vi "write shared memory.vi"(6 "channel classification":T1, 8 "error in":errorcluster, 10 "data table":T2, 11 "module in":refnum<class "Shared Memory runtime.lvclass">) -> (0 "error out":errorcluster, 2 "data table out":T2, 3 "module out":refnum<class "Shared Memory runtime.lvclass">)   [LabVIEW 2014, in "Shared Memory runtime.lvclass"]
uses:
  Shared Memory runtime.lvclass
  <vilib>/NI/Tag Bus/table/data table.ctl
  <vilib>/NI/Tag Bus Module Framework/channel/channel classification.ctl
  Shared Memory runtime.lvclass/Shared Memory runtime.ctl
  <vilib>/NI/Tag Bus/table/data polymorphs/read many/read Doubles.vi
  <vilib>/NI/NI Linux RT IPC/Shared Memory/Pointer Operations/Write 1D Array DBL.vi
  <vilib>/NI/Tag Bus/table/data polymorphs/read many/read Singles.vi
  <vilib>/NI/NI Linux RT IPC/Shared Memory/Pointer Operations/Write 1D Array SGL.vi
  <vilib>/NI/Tag Bus/table/data polymorphs/read many/read I64s.vi
  <vilib>/NI/NI Linux RT IPC/Shared Memory/Pointer Operations/Write 1D Array I64.vi
  <vilib>/NI/Tag Bus/table/data polymorphs/read many/read I32s.vi
  <vilib>/NI/NI Linux RT IPC/Shared Memory/Pointer Operations/Write 1D Array I32.vi
  <vilib>/NI/Tag Bus/table/data polymorphs/read many/read I16s.vi
  <vilib>/NI/NI Linux RT IPC/Shared Memory/Pointer Operations/Write 1D Array I16.vi
  <vilib>/NI/Tag Bus/table/data polymorphs/read many/read I8s.vi
  <vilib>/NI/NI Linux RT IPC/Shared Memory/Pointer Operations/Write 1D Array I8.vi
  <vilib>/NI/Tag Bus/table/data polymorphs/read many/read U64s.vi
  <vilib>/NI/NI Linux RT IPC/Shared Memory/Pointer Operations/Write 1D Array U64.vi
  <vilib>/NI/Tag Bus/table/data polymorphs/read many/read U32s.vi
  <vilib>/NI/NI Linux RT IPC/Shared Memory/Pointer Operations/Write 1D Array U32.vi
  <vilib>/NI/Tag Bus/table/data polymorphs/read many/read U16s.vi
  <vilib>/NI/NI Linux RT IPC/Shared Memory/Pointer Operations/Write 1D Array U16.vi
  <vilib>/NI/Tag Bus/table/data polymorphs/read many/read U8s.vi
  <vilib>/NI/NI Linux RT IPC/Shared Memory/Pointer Operations/Write 1D Array U8.vi
  <vilib>/NI/Tag Bus/table/data polymorphs/read many/read Booleans.vi
  <vilib>/NI/NI Linux RT IPC/Shared Memory/Pointer Operations/Write 1D Array Boolean.vi
  <vilib>/NI/Tag Bus/table/data polymorphs/read sequential/read sequential Doubles.vi
  <vilib>/NI/Tag Bus/table/data polymorphs/read sequential/read sequential Singles.vi
  <vilib>/NI/Tag Bus/table/data polymorphs/read sequential/read sequential I64s.vi
  <vilib>/NI/Tag Bus/table/data polymorphs/read sequential/read sequential I32s.vi
  <vilib>/NI/Tag Bus/table/data polymorphs/read sequential/read sequential I16s.vi
  <vilib>/NI/Tag Bus/table/data polymorphs/read sequential/read sequential I8s.vi
  <vilib>/NI/Tag Bus/table/data polymorphs/read sequential/read sequential U64s.vi
  <vilib>/NI/Tag Bus/table/data polymorphs/read sequential/read sequential U32s.vi
  <vilib>/NI/Tag Bus/table/data polymorphs/read sequential/read sequential U16s.vi
  <vilib>/NI/Tag Bus/table/data polymorphs/read sequential/read sequential U8s.vi
  <vilib>/NI/Tag Bus/table/data polymorphs/read sequential/read sequential Booleans.vi
  Read input data.vi
  Read processing parameters.vi
  Read processing results.vi
  Read output data.vi
  <vilib>/NI/NI Linux RT IPC/Shared Memory/Classes/Shared Memory/Shared Memory.lvclass
  <vilib>/NI/Tag Bus/table/data table.lvlib
  <vilib>/NI/NI Linux RT IPC/Shared Memory/Linux RT IPC.Shared Memory.lvlib
  <vilib>/NI/Tag Bus Module Framework/channel/TBM channel.lvclass
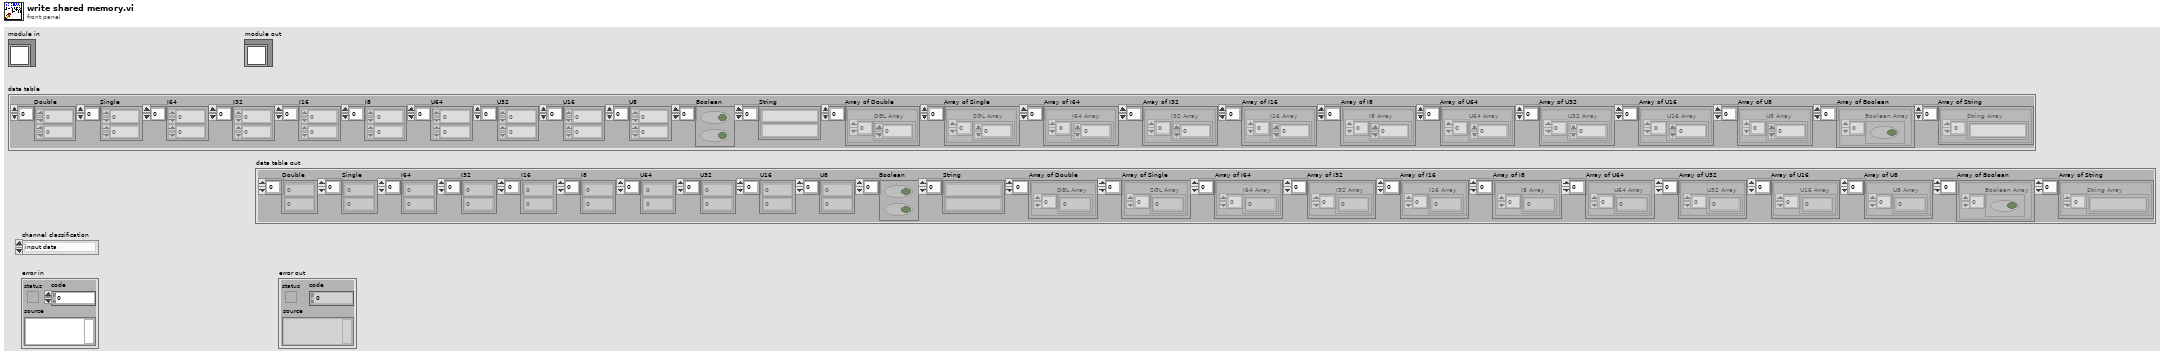
[diagram p1: front panel]
types:
  T1 = typedef "TBM channel.lvclass/channel classification.ctl" = enum16{"input data", "output data", "processing parameter", "processing result"}
  T2 = typedef "tag bus.lvlib/data table.lvlib/data table.ctl" = cluster{"Double":dbl[], "Single":sgl[], "I64":i64[], "I32":i32[], "I16":i16[], "I8":i8[], "U64":u64[], "U32":u32[], "U16":u16[], "U8":u8[], "Boolean":bool[], "String":string[], "Array of Double":cluster{"DBL Array":dbl[]}[], "Array of Single":cluster{"SGL Array":sgl[]}[], "Array of I64":cluster{"I64 Array":i64[]}[], "Array of I32":cluster{"I32 Array":i32[]}[], "Array of I16":cluster{"I16 Array":i16[]}[], "Array of I8":cluster{"I8 Array":i8[]}[], "Array of U64":cluster{"U64 Array":u64[]}[], "Array of U32":cluster{"U32 Array":u32[]}[], "Array of U16":cluster{"U16 Array":u16[]}[], "Array of U8":cluster{"U8 Array":u8[]}[], "Array of Boolean":cluster{"Boolean Array":bool[]}[], "Array of String":cluster{"String Array":string[]}[]}
  T3 = typedef "Shared Memory runtime.lvclass/channel runtime.ctl" = cluster{"channel classification":T1, "data type":T4, "pointer to shared memory":u64, "number of elements":u64, "data dictionary index":cluster{i32[]}, "shared memory":T5, "first tag index":i32, "sequential tags?":bool}
  T4 = typedef "tag bus.lvlib/tag descriptor.lvclass/Data Type.ctl" = enum16{"Double", "Single", "I64", "I32", "I16", "I8", "U64", "U32", "U16", "U8", "Boolean", "String", "Array of Double", "Array of Single", "Array of I64", "Array of I32", "Array of I16", "Array of I8", "Array of U64", "Array of U32", "Array of U16", "Array of U8", "Array of Boolean", "Array of String"}
  T5 = typedef "Linux RT IPC.Shared Memory.lvlib/reference.ctl" = refnum<data-value>
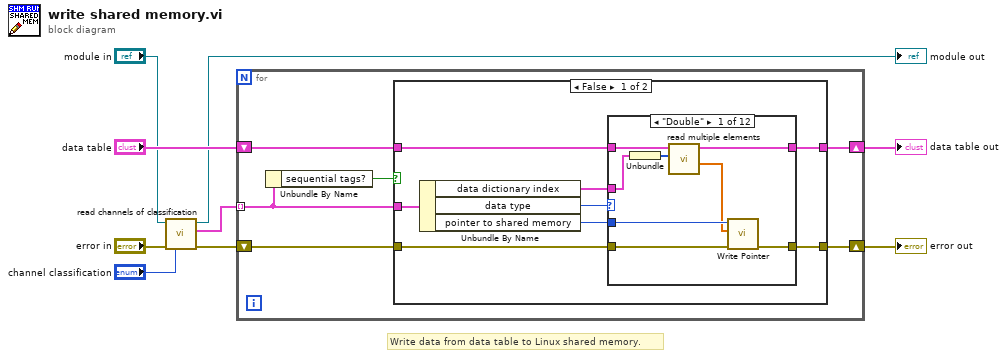
[diagram p0: block diagram]
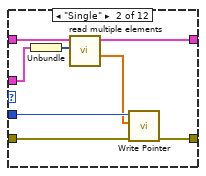
[diagram p2: hidden frame]
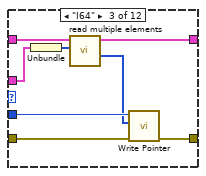
[diagram p3: hidden frame]
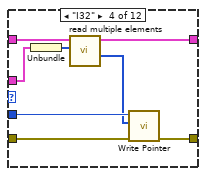
[diagram p4: hidden frame]
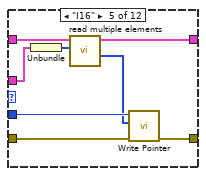
[diagram p5: hidden frame]
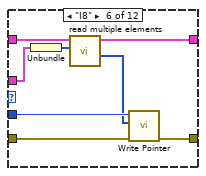
[diagram p6: hidden frame]
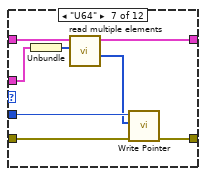
[diagram p7: hidden frame]
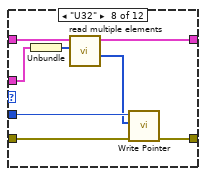
[diagram p8: hidden frame]
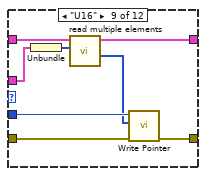
[diagram p9: hidden frame]
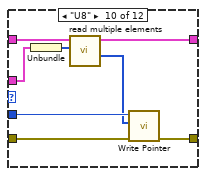
[diagram p10: hidden frame]
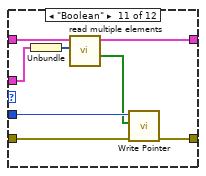
[diagram p11: hidden frame]
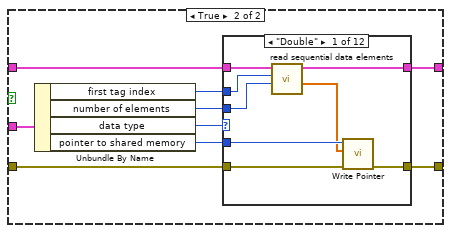
[diagram p13: hidden frame]
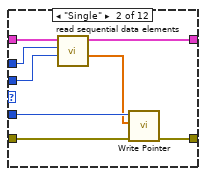
[diagram p14: hidden frame]
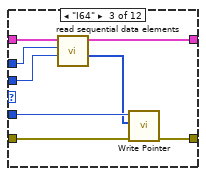
[diagram p15: hidden frame]
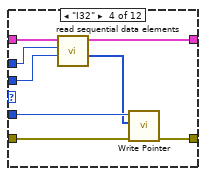
[diagram p16: hidden frame]
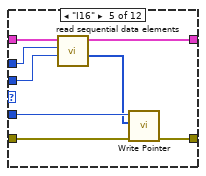
[diagram p17: hidden frame]
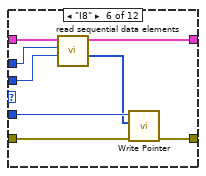
[diagram p18: hidden frame]
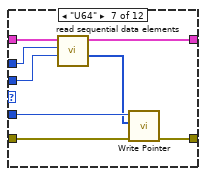
[diagram p19: hidden frame]
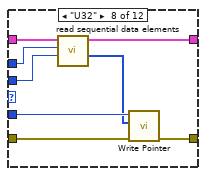
[diagram p20: hidden frame]
diagram:
  # "Write data from data table to Linux shared memory."
  n1 = call "read channels of classification.vi"("channel classification"="channel classification", "error in"="error in", "Shared Memory runtime in"="module in") -> ("error out"=w5:errorcluster, "channels"=w1:T3[], "Shared Memory runtime out"=→"module out":refnum<class "Shared Memory runtime.lvclass">)  [unwired: 6 in]
  n2 = for {
    tunnel: w1 -> [w11] mode=indexing
    shift-right: [w12] -> w8
    shift-left: w5 -> [w13]
    shift-right: [w15] -> w6
    shift-left: "data table" -> [w14]
    # "Write data from data table to Linux shared memory."
    n3 = Unbundle By Name(w11) -> ("sequential tags?"=w10:bool)
    n4 = case shown="False" w10 {
      tunnel: [w17 w122] -> w15
      tunnel: w14 -> [w19 w121]
      tunnel: w13 -> [w20 w120]
      tunnel: [w18 w119] -> w12
      tunnel: w11 -> [w16 w118]
      frame False {
        n5 = Unbundle By Name(w16) -> ("data dictionary index"=w21:cluster{i32[]}, "data type"=w22:T4, "pointer to shared memory"=w23:u64)
        n6 = case shown="\"Double\"" w22 {
          tunnel: w19 -> [w31 w39 w47 w55 w63 w71 w79 w87 w95 w103 w111 w113]
          tunnel: [w30 w38 w46 w54 w62 w70 w78 w86 w94 w102 w110 w113] -> w17
          tunnel: w20 -> [w26 w34 w42 w50 w58 w66 w74 w82 w90 w98 w106 w112]
          tunnel: [w27 w35 w43 w51 w59 w67 w75 w83 w91 w99 w107 w112] -> w18
          tunnel: w23 -> [w25 w33 w41 w49 w57 w65 w73 w81 w89 w97 w105 _]
          tunnel: w21 -> [w29 w37 w45 w53 w61 w69 w77 w85 w93 w101 w109 _]
          frame "Double" {
            n7 = Unbundle(w29) -> (w28:i32[])
            n8 = call-poly <vilib>:"read multiple elements.vi"("indices"=w28, "data table in"=w31) -> ("values"=w24:dbl[], "data table out"=w30:T2)  [unwired: 8 in]
            n9 = call-poly <vilib>:"Write Pointer.vi"("error in (no error)"=w26, "value"=w24, "pointer in"=w25) -> ("error out"=w27:errorcluster)  [unwired: 5 in, 3 out]
          }
          frame "Single" {
            n10 = Unbundle(w37) -> (w36:i32[])
            n11 = call-poly <vilib>:"read multiple elements.vi"("indices"=w36, "data table in"=w39) -> ("values"=w32:sgl[], "data table out"=w38:T2)  [unwired: 8 in]
            n12 = call-poly <vilib>:"Write Pointer.vi"("error in (no error)"=w34, "value"=w32, "pointer in"=w33) -> ("error out"=w35:errorcluster)  [unwired: 5 in, 3 out]
          }
          frame "I64" {
            n13 = Unbundle(w45) -> (w44:i32[])
            n14 = call-poly <vilib>:"read multiple elements.vi"("indices"=w44, "data table in"=w47) -> ("values"=w40:i64[], "data table out"=w46:T2)  [unwired: 8 in]
            n15 = call-poly <vilib>:"Write Pointer.vi"("error in (no error)"=w42, "value"=w40, "pointer in"=w41) -> ("error out"=w43:errorcluster)  [unwired: 5 in, 3 out]
          }
          frame "I32" {
            n16 = Unbundle(w53) -> (w52:i32[])
            n17 = call-poly <vilib>:"read multiple elements.vi"("indices"=w52, "data table in"=w55) -> ("values"=w48:i32[], "data table out"=w54:T2)  [unwired: 8 in]
            n18 = call-poly <vilib>:"Write Pointer.vi"("error in (no error)"=w50, "value"=w48, "pointer in"=w49) -> ("error out"=w51:errorcluster)  [unwired: 5 in, 3 out]
          }
          frame "I16" {
            n19 = Unbundle(w61) -> (w60:i32[])
            n20 = call-poly <vilib>:"read multiple elements.vi"("indices"=w60, "data table in"=w63) -> ("values"=w56:i16[], "data table out"=w62:T2)  [unwired: 8 in]
            n21 = call-poly <vilib>:"Write Pointer.vi"("error in (no error)"=w58, "value"=w56, "pointer in"=w57) -> ("error out"=w59:errorcluster)  [unwired: 5 in, 3 out]
          }
          frame "I8" {
            n22 = Unbundle(w69) -> (w68:i32[])
            n23 = call-poly <vilib>:"read multiple elements.vi"("indices"=w68, "data table in"=w71) -> ("values"=w64:i8[], "data table out"=w70:T2)  [unwired: 8 in]
            n24 = call-poly <vilib>:"Write Pointer.vi"("error in (no error)"=w66, "value"=w64, "pointer in"=w65) -> ("error out"=w67:errorcluster)  [unwired: 5 in, 3 out]
          }
          frame "U64" {
            n25 = Unbundle(w77) -> (w76:i32[])
            n26 = call-poly <vilib>:"read multiple elements.vi"("indices"=w76, "data table in"=w79) -> ("values"=w72:u64[], "data table out"=w78:T2)  [unwired: 8 in]
            n27 = call-poly <vilib>:"Write Pointer.vi"("error in (no error)"=w74, "value"=w72, "pointer in"=w73) -> ("error out"=w75:errorcluster)  [unwired: 5 in, 3 out]
          }
          frame "U32" {
            n28 = Unbundle(w85) -> (w84:i32[])
            n29 = call-poly <vilib>:"read multiple elements.vi"("indices"=w84, "data table in"=w87) -> ("values"=w80:u32[], "data table out"=w86:T2)  [unwired: 8 in]
            n30 = call-poly <vilib>:"Write Pointer.vi"("error in (no error)"=w82, "value"=w80, "pointer in"=w81) -> ("error out"=w83:errorcluster)  [unwired: 5 in, 3 out]
          }
          frame "U16" {
            n31 = Unbundle(w93) -> (w92:i32[])
            n32 = call-poly <vilib>:"read multiple elements.vi"("indices"=w92, "data table in"=w95) -> ("values"=w88:u16[], "data table out"=w94:T2)  [unwired: 8 in]
            n33 = call-poly <vilib>:"Write Pointer.vi"("error in (no error)"=w90, "value"=w88, "pointer in"=w89) -> ("error out"=w91:errorcluster)  [unwired: 5 in, 3 out]
          }
          frame "U8" {
            n34 = Unbundle(w101) -> (w100:i32[])
            n35 = call-poly <vilib>:"read multiple elements.vi"("indices"=w100, "data table in"=w103) -> ("values"=w96:u8[], "data table out"=w102:T2)  [unwired: 8 in]
            n36 = call-poly <vilib>:"Write Pointer.vi"("error in (no error)"=w98, "value"=w96, "pointer in"=w97) -> ("error out"=w99:errorcluster)  [unwired: 5 in, 3 out]
          }
          frame "Boolean" {
            n37 = Unbundle(w109) -> (w108:i32[])
            n38 = call-poly <vilib>:"read multiple elements.vi"("indices"=w108, "data table in"=w111) -> ("values"=w104:bool[], "data table out"=w110:T2)  [unwired: 8 in]
            n39 = call-poly <vilib>:"Write Pointer.vi"("error in (no error)"=w106, "value"=w104, "pointer in"=w105) -> ("error out"=w107:errorcluster)  [unwired: 5 in, 3 out]
          }
          frame Default {
          }
        }
      }
      frame True {
        n40 = Unbundle By Name(w118) -> ("first tag index"=w115:i32, "number of elements"=w114:u64, "data type"=w116:T4, "pointer to shared memory"=w117:u64)
        n41 = case shown="\"Double\"" w116 {
          tunnel: w121 -> [w130 w138 w146 w154 w162 w170 w178 w186 w194 w202 w210 w212]
          tunnel: [w129 w137 w145 w153 w161 w169 w177 w185 w193 w201 w209 w212] -> w122
          tunnel: w120 -> [w125 w133 w141 w149 w157 w165 w173 w181 w189 w197 w205 w211]
          tunnel: [w126 w134 w142 w150 w158 w166 w174 w182 w190 w198 w206 w211] -> w119
          tunnel: w117 -> [w124 w132 w140 w148 w156 w164 w172 w180 w188 w196 w204 _]
          tunnel: w115 -> [w128 w136 w144 w152 w160 w168 w176 w184 w192 w200 w208 _]
          tunnel: w114 -> [w127 w135 w143 w151 w159 w167 w175 w183 w191 w199 w207 _]
          frame "Double" {
            n42 = call-poly <vilib>:"read sequential data elements.vi"("length"=w127, "index"=w128, "data table in"=w130) -> ("values"=w123:dbl[], "data table out"=w129:T2)  [unwired: 7 in]
            n43 = call-poly <vilib>:"Write Pointer.vi"("error in (no error)"=w125, "value"=w123, "pointer in"=w124) -> ("error out"=w126:errorcluster)  [unwired: 5 in, 3 out]
          }
          frame "Single" {
            n44 = call-poly <vilib>:"read sequential data elements.vi"("length"=w135, "index"=w136, "data table in"=w138) -> ("values"=w131:sgl[], "data table out"=w137:T2)  [unwired: 7 in]
            n45 = call-poly <vilib>:"Write Pointer.vi"("error in (no error)"=w133, "value"=w131, "pointer in"=w132) -> ("error out"=w134:errorcluster)  [unwired: 5 in, 3 out]
          }
          frame "I64" {
            n46 = call-poly <vilib>:"read sequential data elements.vi"("length"=w143, "index"=w144, "data table in"=w146) -> ("values"=w139:i64[], "data table out"=w145:T2)  [unwired: 7 in]
            n47 = call-poly <vilib>:"Write Pointer.vi"("error in (no error)"=w141, "value"=w139, "pointer in"=w140) -> ("error out"=w142:errorcluster)  [unwired: 5 in, 3 out]
          }
          frame "I32" {
            n48 = call-poly <vilib>:"read sequential data elements.vi"("length"=w151, "index"=w152, "data table in"=w154) -> ("values"=w147:i32[], "data table out"=w153:T2)  [unwired: 7 in]
            n49 = call-poly <vilib>:"Write Pointer.vi"("error in (no error)"=w149, "value"=w147, "pointer in"=w148) -> ("error out"=w150:errorcluster)  [unwired: 5 in, 3 out]
          }
          frame "I16" {
            n50 = call-poly <vilib>:"read sequential data elements.vi"("length"=w159, "index"=w160, "data table in"=w162) -> ("values"=w155:i16[], "data table out"=w161:T2)  [unwired: 7 in]
            n51 = call-poly <vilib>:"Write Pointer.vi"("error in (no error)"=w157, "value"=w155, "pointer in"=w156) -> ("error out"=w158:errorcluster)  [unwired: 5 in, 3 out]
          }
          frame "I8" {
            n52 = call-poly <vilib>:"read sequential data elements.vi"("length"=w167, "index"=w168, "data table in"=w170) -> ("values"=w163:i8[], "data table out"=w169:T2)  [unwired: 7 in]
            n53 = call-poly <vilib>:"Write Pointer.vi"("error in (no error)"=w165, "value"=w163, "pointer in"=w164) -> ("error out"=w166:errorcluster)  [unwired: 5 in, 3 out]
          }
          frame "U64" {
            n54 = call-poly <vilib>:"read sequential data elements.vi"("length"=w175, "index"=w176, "data table in"=w178) -> ("values"=w171:u64[], "data table out"=w177:T2)  [unwired: 7 in]
            n55 = call-poly <vilib>:"Write Pointer.vi"("error in (no error)"=w173, "value"=w171, "pointer in"=w172) -> ("error out"=w174:errorcluster)  [unwired: 5 in, 3 out]
          }
          frame "U32" {
            n56 = call-poly <vilib>:"read sequential data elements.vi"("length"=w183, "index"=w184, "data table in"=w186) -> ("values"=w179:u32[], "data table out"=w185:T2)  [unwired: 7 in]
            n57 = call-poly <vilib>:"Write Pointer.vi"("error in (no error)"=w181, "value"=w179, "pointer in"=w180) -> ("error out"=w182:errorcluster)  [unwired: 5 in, 3 out]
          }
          frame "U16" {
            n58 = call-poly <vilib>:"read sequential data elements.vi"("length"=w191, "index"=w192, "data table in"=w194) -> ("values"=w187:u16[], "data table out"=w193:T2)  [unwired: 7 in]
            n59 = call-poly <vilib>:"Write Pointer.vi"("error in (no error)"=w189, "value"=w187, "pointer in"=w188) -> ("error out"=w190:errorcluster)  [unwired: 5 in, 3 out]
          }
          frame "U8" {
            n60 = call-poly <vilib>:"read sequential data elements.vi"("length"=w199, "index"=w200, "data table in"=w202) -> ("values"=w195:u8[], "data table out"=w201:T2)  [unwired: 7 in]
            n61 = call-poly <vilib>:"Write Pointer.vi"("error in (no error)"=w197, "value"=w195, "pointer in"=w196) -> ("error out"=w198:errorcluster)  [unwired: 5 in, 3 out]
          }
          frame "Boolean" {
            n62 = call-poly <vilib>:"read sequential data elements.vi"("length"=w207, "index"=w208, "data table in"=w210) -> ("values"=w203:bool[], "data table out"=w209:T2)  [unwired: 7 in]
            n63 = call-poly <vilib>:"Write Pointer.vi"("error in (no error)"=w205, "value"=w203, "pointer in"=w204) -> ("error out"=w206:errorcluster)  [unwired: 5 in, 3 out]
          }
          frame Default {
          }
        }
      }
    }
  }
  "error out" <- w8
  "data table out" <- w6
